vi "Write CommandConstruction.vi"(10 "CommandConstruction.lvclass":refnum<class "CommandConstruction.lvclass">, 11 "SALCommunicator in":refnum<class "SALCommunicatorDL.lvclass">) -> (3 "SALCommunicator out":refnum<class "SALCommunicatorDL.lvclass">)   [LabVIEW 2016, in "SALCommunicatorDL.lvclass"]
uses:
  SALCommunicatorDL.lvclass
  CommandConstruction/CommandConstruction.lvclass
  SALCommunicatorDL.lvclass/SALCommunicatorDL.ctl
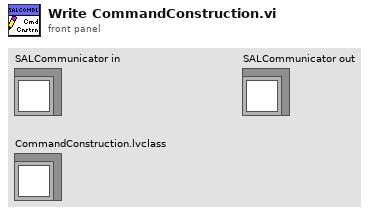
[diagram p1: front panel]
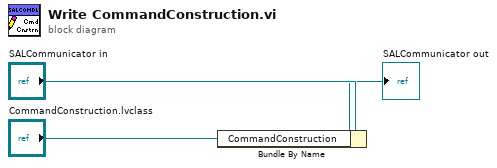
[diagram p0: block diagram]
diagram:
  n1 = Bundle By Name(cluster="SALCommunicator in", "CommandConstruction"="CommandConstruction.lvclass") -> (→"SALCommunicator out":refnum<class "SALCommunicatorDL.lvclass">)
